vi "Begin.vi"(11 "Image Size":T1=enum."160x120") -> (0 "error out":errorcluster)   [LabVIEW 2011]
doc: "Called before other user functions, this VI is expected to open initial I/O refnums, load in file data, and do all program initialization. Notice that the <B>error out</B> terminal is simply used for data flow. Wiring it to other structures or subVIs ensures that this VI runs first."
uses:
  <vilib>/Rock Robotics/WPI/Camera/WPI_CameraImageSize.ctl
  <vilib>/Rock Robotics/WPI/Camera/WPI_CameraExposure Values.ctl
  <vilib>/Rock Robotics/WPI/Camera/WPI_CameraFrameRate.ctl
  <vilib>/Rock Robotics/WPI/Camera/WPI_CameraWhite Balance Values.ctl
  <vilib>/Rock Robotics/SystemInterfaces/DIO/FPGA_DIOPWMChannel.ctl
  <vilib>/Rock Robotics/SystemInterfaces/DIO/FPGA_DIOChannel.ctl
  <vilib>/Rock Robotics/WPI/Encoder/WPI_EncoderType.ctl
  <vilib>/Rock Robotics/SystemInterfaces/Typedef/FPGA_TypedefAnalogModule.ctl
  <vilib>/Rock Robotics/SystemInterfaces/AI/FPGA_AIChannel.ctl
  <vilib>/Rock Robotics/SystemInterfaces/Typedef/FPGA_TypedefDigitalModule.ctl
  <vilib>/Rock Robotics/SystemInterfaces/DIO/FPGA_DIORelayChannel.ctl
  <vilib>/Rock Robotics/WPI/Joystick/WPI_JoystickDeviceEnum.ctl
  <vilib>/Rock Robotics/SystemInterfaces/Typedef/FPGA_TypedefSolenoidModule.ctl
  <vilib>/Rock Robotics/WPI/Solenoid/WPI_SolenoidChannel.ctl
  <vilib>/Rock Robotics/WPI/Relay/WPI_RelayDirection.ctl
  <vilib>/Rock Robotics/WPI/RobotDrive/WPI_RobotDriveOpen4MotorWithVictor.vi
  <vilib>/Rock Robotics/WPI/MotorControl/WPI_MotorControlOpen Victor.vi
  <vilib>/Rock Robotics/WPI/Counter/WPI_CounterDigitalInputToDigitalSource.vi
  <vilib>/Rock Robotics/WPI/Counter/WPI_CounterOpen Gear Tooth Sensor Mode.vi
  <vilib>/Rock Robotics/WPI/Solenoid/WPI_SolenoidOpenDouble.vi
  <vilib>/Rock Robotics/WPI/Compressor/WPI_CompressorGetSetRefNum.vi
panel:
  in  "Image Size 2":T1=enum."160x120"
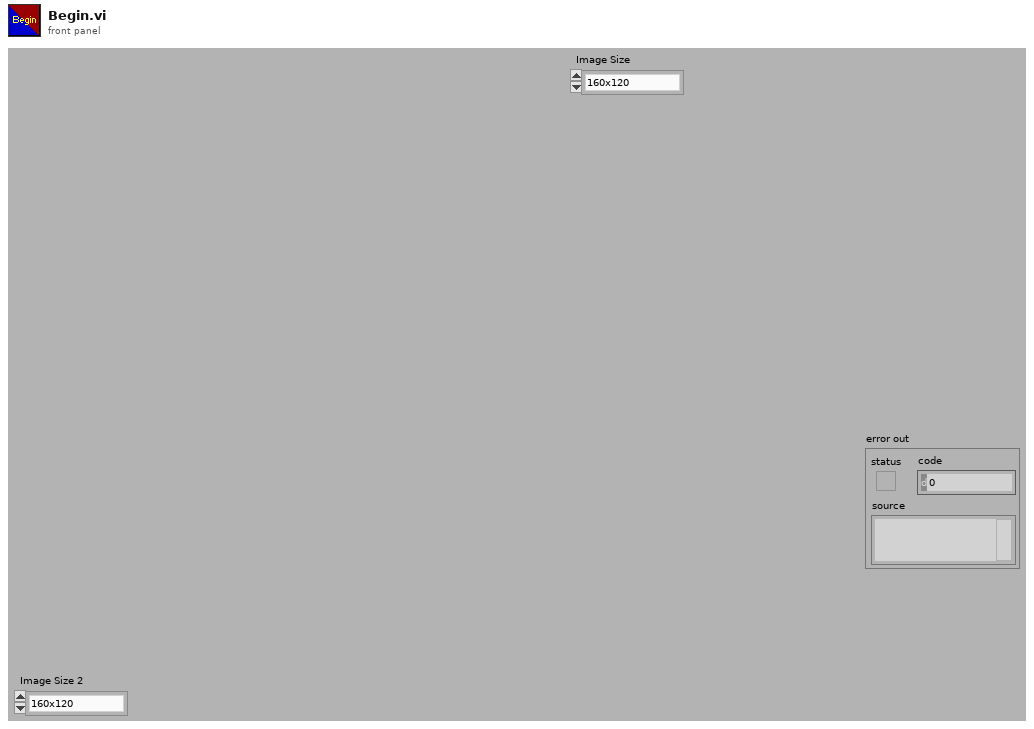
[diagram p1: front panel]
types:
  T1 = typedef "WPI_CameraImageSize.ctl" = enum16{"640x480", "320x240", "160x120"}
  T2 = typedef "WPI_RelayDirection.ctl" = enum16{"Both directions", "Forward only", "Reverse only"}
  T3 = typedef "FPGA_DIORelayChannel.ctl" = enum8{"Relay 1", "Relay 2", "Relay 3", "Relay 4", "Relay 5", "Relay 6", "Relay 7", "Relay 8", "Invalid"}
  T4 = typedef "FPGA_TypedefDigitalModule.ctl" = enum16{"Digital Module 1", "Digital Module 2"}
  T5 = typedef "WPI_SolenoidChannel.ctl" = enum8{"Solenoid 1", "Solenoid 2", "Solenoid 3", "Solenoid 4", "Solenoid 5", "Solenoid 6", "Solenoid 7", "Solenoid 8", "Invalid"}
  T6 = typedef "FPGA_TypedefSolenoidModule.ctl" = enum16{"Solenoid Module 1", "Solenoid Module 2"}
  T7 = typedef "FPGA_DIOChannel.ctl" = enum8{"DIO 1", "DIO 2", "DIO 3", "DIO 4", "DIO 5", "DIO 6", "DIO 7", "DIO 8", "DIO 9", "DIO 10", "DIO 11", "DIO 12", "DIO 13", "DIO 14", "Invalid"}
  T8 = typedef "WPI_JoystickDeviceEnum.ctl" = enum16{"USB 1", "USB 2", "USB 3", "USB 4", "Kinect 1", "Kinect 2"}
  T9 = typedef "FPGA_DIOPWMChannel.ctl" = enum8{"PWM 1", "PWM 2", "PWM 3", "PWM 4", "PWM 5", "PWM 6", "PWM 7", "PWM 8", "PWM 9", "PWM 10", "Invalid"}
  T10 = typedef "FPGA_AIChannel.ctl" = enum8{"AI 1", "AI 2", "AI 3", "AI 4", "AI 5", "AI 6", "AI 7", "AI 8", "Invalid"}
  T11 = typedef "FPGA_TypedefAnalogModule.ctl" = enum16{"Analog Module 1", "Analog Module 2"}
  T12 = typedef "WPI_EncoderType.ctl" = enum16{"1x", "2x", "4x"}
  T13 = typedef "WPI_CameraFrameRate.ctl" = u32
  T14 = typedef "WPI_CameraExposure Values.ctl" = enum16{"Auto", "Flicker-free 50 Hz", "Flicker-free 60 Hz", "Hold current"}
  T15 = typedef "WPI_CameraWhite Balance Values.ctl" = enum16{"Auto", "Fixed indoor", "Fixed outdoor 1", "Fixed outdoor 2", "Fixed fluorescent 1", "Fixed fluorescent 2", "Hold current"}
  T16 = typedef "WPI_MotorControlDeviceRef.ctl" = cluster{"DeviceStatus":errorcluster, "Type":enum16{"PWM", "CAN"}, "PWM":cluster{"Digital Module":T4, "PWM Channel":T9, "DeadBand":T17}, "CAN":cluster{"Device Number":u8, "Control Mode":T18, "Semaphore":T19, "Max Vout":dbl}, "Invert":bool, "TransformRef":T20, "InvTransformRef":T20}
  T17 = typedef "WPI_PWMDeadband.ctl" = cluster{"Name":string, "maxPositivePwm":i32, "minPositivePwm":i32, "centerPwm":i32, "maxNegativePwm":i32, "minNegativePwm":i32, "angularRange":u16}
  T18 = typedef "WPI_CANJaguar_ControlMode.ctl" = enum8{"Percent VBus", "Current", "Speed", "Position", "Voltage"}
  T19 = typedef "Semaphore RefNum" = refnum<k1>
  T20 = typedef "WPI_PWMTransform_ConPane.ctl" = refnum<vi>
  T21 = typedef "WPI_RobotDriveDevRef.ctl" = cluster{"DevStatus":errorcluster, "Motors[]":T16[], "Square Inputs":bool, "Max Output":dbl, "Isochronous":bool}
  T22 = typedef "WPI_CameraDevRef.ctl" = cluster{"Camera Address":string, "CameraStatus":errorcluster, "Acquire Image Notifier":refnum<notifier>}
  T23 = typedef "WPI_DigitalInputDevRef.ctl" = cluster{"DevStatus":errorcluster, "DIO Channel":T7, "Digital Module":T4}
  T24 = typedef "WPI_JoystickDevRef.ctl" = cluster{"Device":T8}
  T25 = typedef "WPI_AnalogChannelDevRef.ctl" = cluster{"DevStatus":errorcluster, "Analog Module":T11, "Analog Channel":T10}
  T26 = typedef "WPI_RelayDevRef.ctl" = cluster{"DevStatus":errorcluster, "Relay Channel":T3, "Digital Module":T4, "Relay Direction":T2}
  T27 = typedef "FPGA_CounterEncoderSourceConvertionLVSourceType.ctl" = cluster{"DevStatus":errorcluster, "AnalogTriggerMode?":bool, "DigitalMode":cluster{"Digital Module":T4, "DIO Channel":T28}, "AnalogTriggerMode":cluster{"AnalogTriggerIndex":T29, "OutputType":T30}}
  T28 = typedef "FPGA_DIODigitalSourceChannel.ctl" = enum8{"DIO 1", "DIO 2", "DIO 3", "DIO 4", "DIO 5", "DIO 6", "DIO 7", "DIO 8", "DIO 9", "DIO 10", "DIO 11", "DIO 12", "DIO 13", "DIO 14", "Disabled"}
  T29 = typedef "FPGA_AnalogTriggerIndex.ctl" = enum8{"Trig 0", "Trig 1", "Trig 2", "Trig 3", "Trig 4", "Trig 5", "Trig 6", "Trig 7", "Invalid"}
  T30 = typedef "FPGA_AnalogTriggerOutType.ctl" = enum16{"InWindow", "TriggerState", "Rising", "Falling"}
  T31 = typedef "WPI_EncoderDevRef.ctl" = cluster{"DevStatus":errorcluster, "EncoderIndex":T32, "CounterIndex":T33, "DistancePerCount":dbl, "Decoding Type":T12}
  T32 = typedef "FPGA_EncoderIdx.ctl" = enum8{"Enc 0", "Enc 1", "Enc 2", "Enc 3", "Invalid"}
  T33 = typedef "FPGA_CounterCtrSystemIndex.ctl" = enum8{"Ctr 0", "Ctr 1", "Ctr 2", "Ctr 3", "Ctr 4", "Ctr 5", "Ctr 6", "Ctr 7", "Invalid"}
  T34 = typedef "WPI_SolenoidDevRef.ctl" = cluster{"DevStatus":errorcluster, "Solenoid Module":T6, "Forward Solenoid Channel":T5, "Reverse Solenoid Channel":T5}
  T35 = typedef "WPI_CompressorDevRef.ctl" = cluster{"DevStatus":errorcluster, "DigitalInputDevRef":T23, "RelayDevRef":T26}
  T36 = typedef "WPI_CounterDevRef.ctl" = cluster{"DevStatus":errorcluster, "CntIndex":T33}
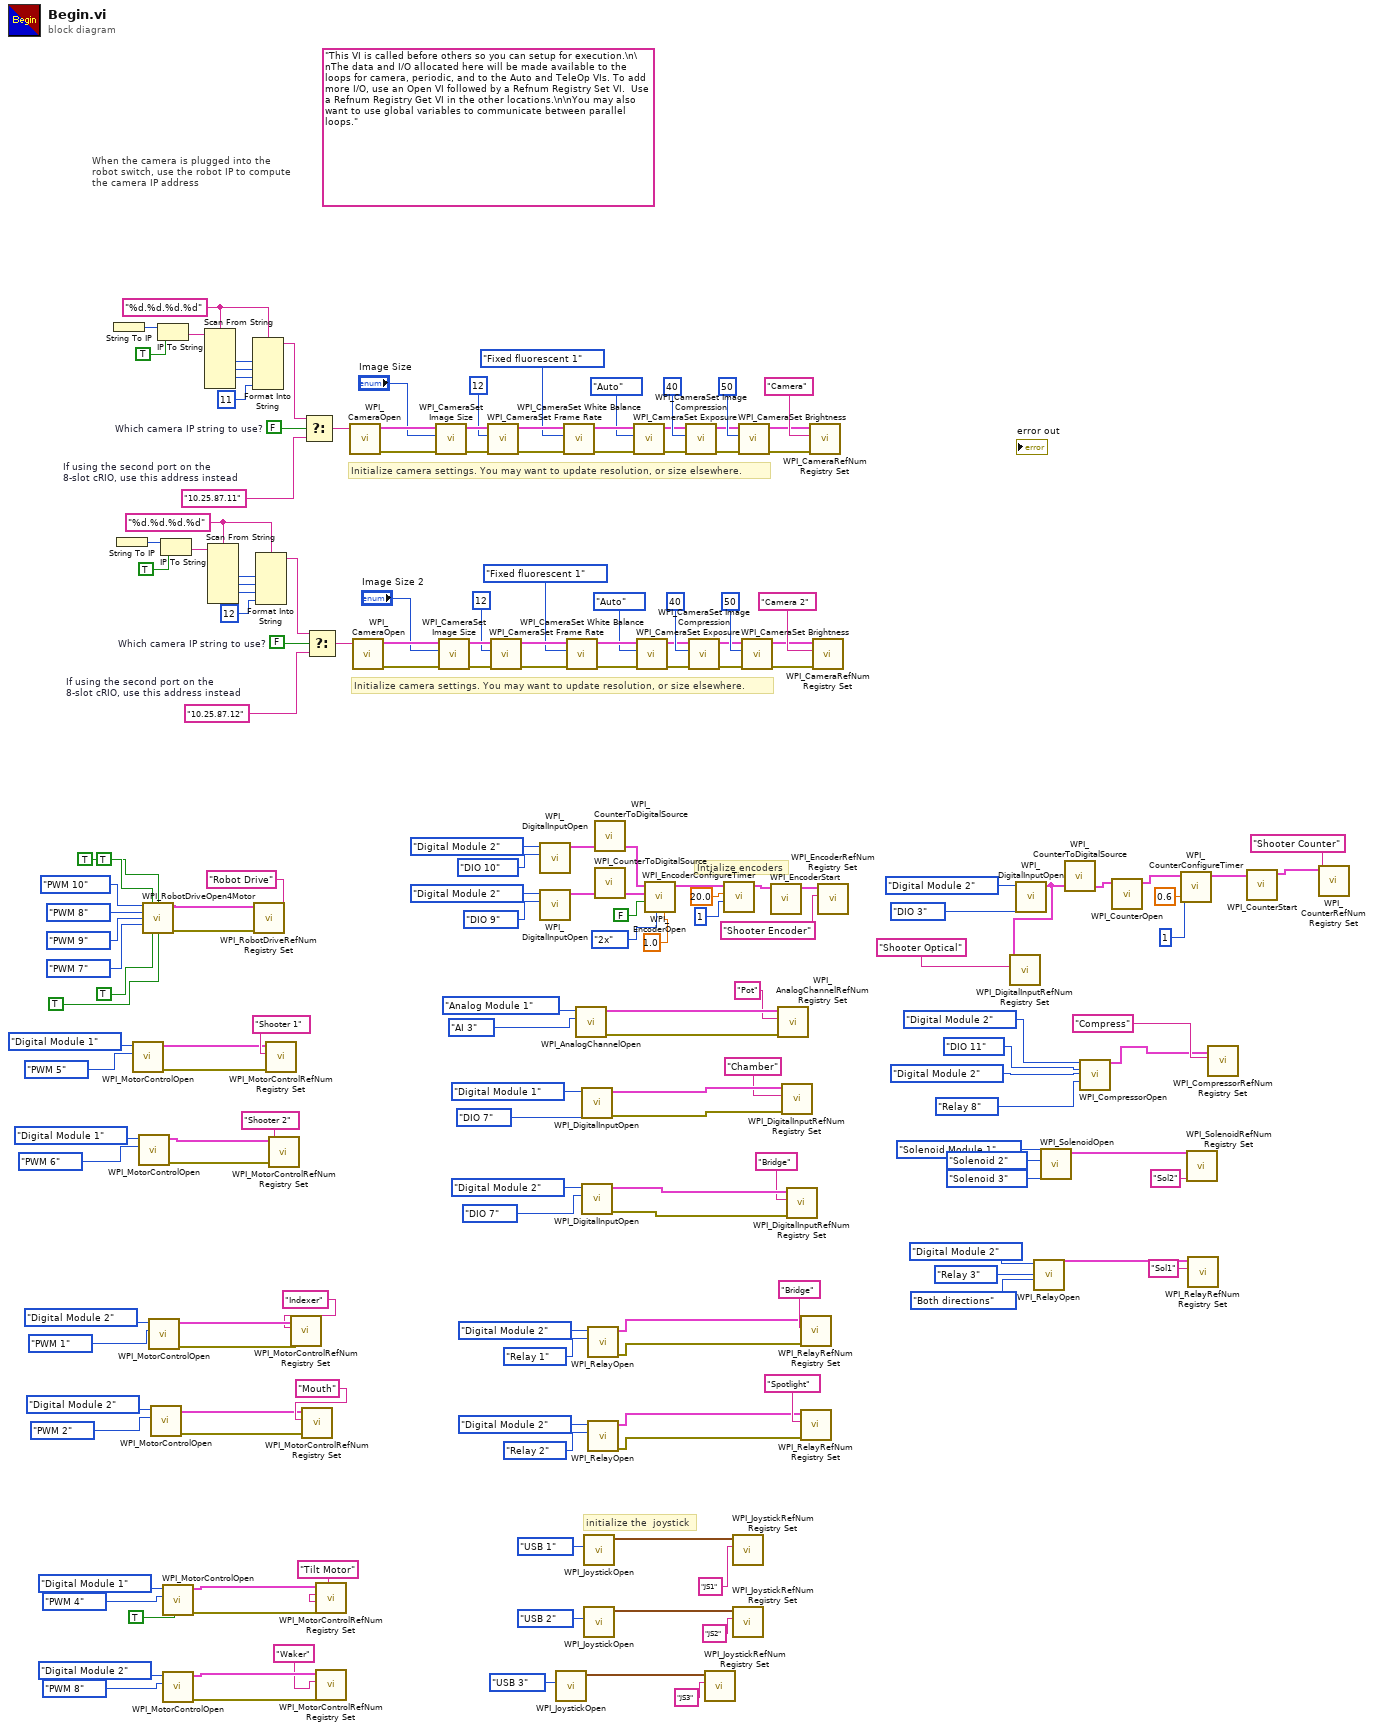
[diagram p0: block diagram]
diagram:
  w121 = FALSE  # Which camera IP string to use?
  w125 = "%d.%d.%d.%d" ("format string")
  w122 = "10.25.87.12"  # If using the second port on the 8-slot cRIO, use this address instead
  w154 = FALSE  # Which camera IP string to use?
  w158 = "%d.%d.%d.%d" ("format string")
  (unwired) "This VI is called before others so you can setup for execution.\n\nThe data and I/O allocated here will be made available to the loops for camera, periodic, and to the Auto and TeleOp VIs. To add more I/O, use an Open VI followed by a Refnum Registry Set VI.  Use a Refnum Registry Get VI in the other locations.\n\nYou may also want to use global variables to communicate between parallel loops."
  w155 = "10.25.87.11"  # If using the second port on the 8-slot cRIO, use this address instead
  # "initialize the  joystick"
  # "Intialize encoders"
  # "Initialize camera settings. You may want to update resolution, or size elsewhere."
  # "When the camera is plugged into the\nrobot switch, use the robot IP to compute\nthe camera IP address"
  # "Initialize camera settings. You may want to update resolution, or size elsewhere."
  n1 = String To IP() -> (0:w165:u32)  [unwired: 1 in]
  n2 = String To IP() -> (0:w132:u32)  [unwired: 1 in]
  n3 = call-poly <vilib>:"WPI_MotorControlOpen.vi"("PWM Channel"=FPGA_DIOPWMChannel."PWM 5", "Digital Module (Module 1)"=FPGA_TypedefDigitalModule."Digital Module 1") -> ("error out"=w104:errorcluster, "MotorControlDeviceRef"=w105:T16)  [unwired: 8 in]
  n4 = call-poly <vilib>:"WPI_MotorControlOpen.vi"("PWM Channel"=FPGA_DIOPWMChannel."PWM 6", "Digital Module (Module 1)"=FPGA_TypedefDigitalModule."Digital Module 1") -> ("error out"=w102:errorcluster, "MotorControlDeviceRef"=w103:T16)  [unwired: 8 in]
  n5 = call-poly <vilib>:"WPI_RobotDriveOpen4Motor.vi"("Rear Left Motor"=FPGA_DIOPWMChannel."PWM 10", "Rear Left Motor Inverted"=TRUE, "Rear Right Motor Inverted"=TRUE, "Rear Right Motor"=FPGA_DIOPWMChannel."PWM 8", "Front Left Motor"=FPGA_DIOPWMChannel."PWM 9", "Front Right Motor"=FPGA_DIOPWMChannel."PWM 7", "Front Left Motor Inverted"=TRUE, "Front Right Motor Inverted"=TRUE) -> ("RobotDriveDevRef"=w47:T21, "error out"=w46:errorcluster)  [unwired: 6 in]
  n6 = call-poly <vilib>:"WPI_MotorControlOpen.vi"("PWM Channel"=FPGA_DIOPWMChannel."PWM 1", "Digital Module (Module 1)"=FPGA_TypedefDigitalModule."Digital Module 2") -> ("error out"=w55:errorcluster, "MotorControlDeviceRef"=w56:T16)  [unwired: 8 in]
  n7 = call-poly <vilib>:"WPI_MotorControlOpen.vi"("PWM Channel"=FPGA_DIOPWMChannel."PWM 2", "Digital Module (Module 1)"=FPGA_TypedefDigitalModule."Digital Module 2") -> ("error out"=w97:errorcluster, "MotorControlDeviceRef"=w98:T16)  [unwired: 8 in]
  n8 = IP To String(1:TRUE ("dot notation? (F)"), 2:w165) -> (0:w163:string)
  n9 = IP To String(1:TRUE ("dot notation? (F)"), 2:w132) -> (0:w130:string)
  n10 = call-poly <vilib>:"WPI_MotorControlOpen.vi"("Invert"=TRUE, "PWM Channel"=FPGA_DIOPWMChannel."PWM 4", "Digital Module (Module 1)"=FPGA_TypedefDigitalModule."Digital Module 1") -> ("error out"=w91:errorcluster, "MotorControlDeviceRef"=w92:T16)  [unwired: 7 in]
  n11 = call-poly <vilib>:"WPI_MotorControlOpen.vi"("PWM Channel"=FPGA_DIOPWMChannel."PWM 8", "Digital Module (Module 1)"=FPGA_TypedefDigitalModule."Digital Module 2") -> ("error out"=w35:errorcluster, "MotorControlDeviceRef"=w34:T16)  [unwired: 8 in]
  n12 = Scan From String(format string=w158, input string=w163) -> (output 1=w162:i32, output 2=w161:i32, output 3=w160:i32)  [unwired: 7 in, 3 out]
  n13 = Scan From String(format string=w125, input string=w130) -> (output 1=w129:i32, output 2=w128:i32, output 3=w127:i32)  [unwired: 7 in, 3 out]
  n14 = Format Into String(format string=w158, w162, w161, w160, 11 ("Compression")) -> (resulting string=w156:string)  [unwired: 2 in, 1 out]
  n15 = call <vilib>:"WPI_RobotDriveRefNum Registry Set.vi"("error in (no error)"=w46, "refnum name"="Robot Drive", "RobotDriveDevRef"=w47) -> ()  [unwired: 7 in, 2 out]
  n16 = Format Into String(format string=w125, w129, w128, w127, 12 ("Compression")) -> (resulting string=w123:string)  [unwired: 2 in, 1 out]
  n17 = call <vilib>:"WPI_MotorControlRefNum Registry Set.vi"("error in (no error)"=w104, "refnum name"="Shooter 1", "MotorControlDevRef"=w105) -> ()  [unwired: 7 in, 2 out]
  n18 = call <vilib>:"WPI_MotorControlRefNum Registry Set.vi"("error in (no error)"=w102, "refnum name"="Shooter 2", "MotorControlDevRef"=w103) -> ()  [unwired: 7 in, 2 out]
  n19 = call <vilib>:"WPI_MotorControlRefNum Registry Set.vi"("error in (no error)"=w55, "refnum name"="Indexer", "MotorControlDevRef"=w56) -> ()  [unwired: 7 in, 2 out]
  n20 = call <vilib>:"WPI_MotorControlRefNum Registry Set.vi"("error in (no error)"=w97, "refnum name"="Mouth", "MotorControlDevRef"=w98) -> ()  [unwired: 7 in, 2 out]
  n21 = Select(t=w156, s=w154, f=w155) -> (s? t:f=w157:string)
  n22 = Select(t=w123, s=w121, f=w122) -> (s? t:f=w124:string)
  n23 = call <vilib>:"WPI_MotorControlRefNum Registry Set.vi"("error in (no error)"=w91, "refnum name"="Tilt Motor", "MotorControlDevRef"=w92) -> ()  [unwired: 7 in, 2 out]
  n24 = call <vilib>:"WPI_MotorControlRefNum Registry Set.vi"("error in (no error)"=w35, "refnum name"="Waker", "MotorControlDevRef"=w34) -> ()  [unwired: 7 in, 2 out]
  n25 = call <vilib>:"WPI_CameraOpen.vi"("Camera Address"=w157) -> ("error out"=w177:errorcluster, "CameraDevRef"=w178:T22)  [unwired: 1 in, 8 out]
  n26 = call <vilib>:"WPI_CameraOpen.vi"("Camera Address"=w124) -> ("error out"=w144:errorcluster, "CameraDevRef"=w145:T22)  [unwired: 1 in, 8 out]
  n27 = call <vilib>:"WPI_CameraSet Image Size.vi"("error in (no error)"=w177, "Image Size"="Image Size", "CameraDevRef"=w178) -> ("error out"=w176:errorcluster, "CameraDevRef Out"=w179:T22)  [unwired: 7 out]
  n28 = call <vilib>:"WPI_CameraSet Image Size.vi"("error in (no error)"=w144, "Image Size"="Image Size 2", "CameraDevRef"=w145) -> ("error out"=w143:errorcluster, "CameraDevRef Out"=w146:T22)  [unwired: 7 out]
  n29 = call <vilib>:"WPI_CameraSet Frame Rate.vi"("error in (no error)"=w176, "Frame Rate (fps)"=T13 12, "CameraDevRef"=w179) -> ("error out"=w175:errorcluster, "CameraDevRef Out"=w181:T22)  [unwired: 7 out]
  n30 = call <vilib>:"WPI_CameraSet Frame Rate.vi"("error in (no error)"=w143, "Frame Rate (fps)"=T13 12, "CameraDevRef"=w146) -> ("error out"=w142:errorcluster, "CameraDevRef Out"=w148:T22)  [unwired: 7 out]
  n31 = call <vilib>:"WPI_DigitalInputOpen.vi"("DIO Channel"=FPGA_DIOChannel."DIO 10", "Digital Module (Module 1)"=FPGA_TypedefDigitalModule."Digital Module 2") -> ("DigitalInputDevRef"=w88:T23)  [unwired: 8 in, 1 out]
  n32 = call <vilib>:"WPI_DigitalInputOpen.vi"("DIO Channel"=FPGA_DIOChannel."DIO 9", "Digital Module (Module 1)"=FPGA_TypedefDigitalModule."Digital Module 2") -> ("DigitalInputDevRef"=w84:T23)  [unwired: 8 in, 1 out]
  n33 = call <vilib>:"WPI_JoystickOpen.vi"("JoystickDevice"=WPI_JoystickDeviceEnum."USB 3") -> ("JoystickDevRef"=w19:T24)  [unwired: 10 out]
  n34 = call <vilib>:"WPI_CameraSet White Balance.vi"("error in (no error)"=w175, "White Balance"=WPI_CameraWhite_Balance_Values."Fixed fluorescent 1", "CameraDevRef"=w181) -> ("error out"=w174:errorcluster, "CameraDevRef Out"=w180:T22)  [unwired: 7 out]
  n35 = call <vilib>:"WPI_CameraSet White Balance.vi"("error in (no error)"=w142, "White Balance"=WPI_CameraWhite_Balance_Values."Fixed fluorescent 1", "CameraDevRef"=w148) -> ("error out"=w141:errorcluster, "CameraDevRef Out"=w147:T22)  [unwired: 7 out]
  n36 = call <vilib>:"WPI_AnalogChannelOpen.vi"("Analog Channel"=FPGA_AIChannel."AI 3", "Analog Module (Module 1)"=FPGA_TypedefAnalogModule."Analog Module 1") -> ("error out"=w69:errorcluster, "AIDeviceRef"=w71:T25)  [unwired: 8 in]
  n37 = call <vilib>:"WPI_DigitalInputOpen.vi"("DIO Channel"=FPGA_DIOChannel."DIO 7", "Digital Module (Module 1)"=FPGA_TypedefDigitalModule."Digital Module 1") -> ("error out"=w64:errorcluster, "DigitalInputDevRef"=w66:T23)  [unwired: 8 in]
  n38 = call <vilib>:"WPI_DigitalInputOpen.vi"("DIO Channel"=FPGA_DIOChannel."DIO 7", "Digital Module (Module 1)"=FPGA_TypedefDigitalModule."Digital Module 2") -> ("error out"=w36:errorcluster, "DigitalInputDevRef"=w38:T23)  [unwired: 8 in]
  n39 = call <vilib>:"WPI_JoystickOpen.vi"("JoystickDevice"=WPI_JoystickDeviceEnum."USB 1") -> ("JoystickDevRef"=w51:T24)  [unwired: 10 out]
  n40 = call <vilib>:"WPI_JoystickOpen.vi"("JoystickDevice"=WPI_JoystickDeviceEnum."USB 2") -> ("JoystickDevRef"=w50:T24)  [unwired: 10 out]
  n41 = call <vilib>:"WPI_RelayOpen.vi"("Relay Channel"=FPGA_DIORelayChannel."Relay 1", "Digital Module (Module 1)"=FPGA_TypedefDigitalModule."Digital Module 2") -> ("error out"=w41:errorcluster, "RelayDevRef"=w42:T26)  [unwired: 8 in]
  n42 = call <vilib>:"WPI_RelayOpen.vi"("Relay Channel"=FPGA_DIORelayChannel."Relay 2", "Digital Module (Module 1)"=FPGA_TypedefDigitalModule."Digital Module 2") -> ("error out"=w59:errorcluster, "RelayDevRef"=w60:T26)  [unwired: 8 in]
  n43 = call-poly <vilib>:"WPI_CounterToDigitalSource.vi"("DigitalInputDevRef"=w88) -> ("Digital Source"=w87:T27)  [unwired: 6 in]
  n44 = call-poly <vilib>:"WPI_CounterToDigitalSource.vi"("DigitalInputDevRef"=w84) -> ("Digital Source"=w83:T27)  [unwired: 6 in]
  n45 = call <vilib>:"WPI_CameraSet Exposure.vi"("error in (no error)"=w174, "Exposure"=WPI_CameraExposure_Values."Auto", "CameraDevRef"=w180) -> ("error out"=w173:errorcluster, "CameraDevRef Out"=w183:T22)  [unwired: 7 out]
  n46 = call <vilib>:"WPI_CameraSet Exposure.vi"("error in (no error)"=w141, "Exposure"=WPI_CameraExposure_Values."Auto", "CameraDevRef"=w147) -> ("error out"=w140:errorcluster, "CameraDevRef Out"=w150:T22)  [unwired: 7 out]
  n47 = call <vilib>:"WPI_EncoderOpen.vi"("DistancePerCount"=1.0, "Decoding Type"=WPI_EncoderType."2x", "Invert Direction (False)"=FALSE, "BSource"=w83, "ASource"=w87) -> ("EncoderDevRef"=w81:T31)  [unwired: 5 in, 1 out]
  n48 = call <vilib>:"WPI_CameraSet Image Compression.vi"("error in (no error)"=w173, "Compression"=40, "CameraDevRef"=w183) -> ("error out"=w172:errorcluster, "CameraDevRef Out"=w182:T22)  [unwired: 7 out]
  n49 = call <vilib>:"WPI_CameraSet Image Compression.vi"("error in (no error)"=w140, "Compression"=40, "CameraDevRef"=w150) -> ("error out"=w139:errorcluster, "CameraDevRef Out"=w149:T22)  [unwired: 7 out]
  n50 = call <vilib>:"WPI_JoystickRefNum Registry Set.vi"("refnum name"="JS3", "JoystickDevRef"=w19) -> ()  [unwired: 1 in, 9 out]
  n51 = call <vilib>:"WPI_EncoderConfigureTimer.vi"("Number Samples to Average"=u8 1, "Minimum Rate"=20.0, "EncoderDevRef"=w81) -> ("EncoderDevRef"=w75:T31)  [unwired: 7 in, 1 out]
  n52 = call <vilib>:"WPI_JoystickRefNum Registry Set.vi"("refnum name"="JS1", "JoystickDevRef"=w51) -> ()  [unwired: 1 in, 9 out]
  n53 = call <vilib>:"WPI_JoystickRefNum Registry Set.vi"("refnum name"="JS2", "JoystickDevRef"=w50) -> ()  [unwired: 1 in, 9 out]
  n54 = call <vilib>:"WPI_CameraSet Brightness.vi"("error in (no error)"=w172, "Brightness"=50, "CameraDevRef"=w182) -> ("error out"=w170:errorcluster, "CameraDevRef Out"=w171:T22)  [unwired: 7 out]
  n55 = call <vilib>:"WPI_CameraSet Brightness.vi"("error in (no error)"=w139, "Brightness"=50, "CameraDevRef"=w149) -> ("error out"=w137:errorcluster, "CameraDevRef Out"=w138:T22)  [unwired: 7 out]
  n56 = call <vilib>:"WPI_EncoderStart.vi"("EncoderDevRef"=w75) -> ("EncoderDevRef"=w74:T31)  [unwired: 9 in, 1 out]
  n57 = call <vilib>:"WPI_AnalogChannelRefNum Registry Set.vi"("error in (no error)"=w69, "refnum name"="Pot", "AIDeviceRef"=w71) -> ()  [unwired: 7 in, 2 out]
  n58 = call <vilib>:"WPI_DigitalInputRefNum Registry Set.vi"("error in (no error)"=w64, "refnum name"="Chamber", "DigitalInputDevRef"=w66) -> ()  [unwired: 7 in, 2 out]
  n59 = call <vilib>:"WPI_DigitalInputRefNum Registry Set.vi"("error in (no error)"=w36, "refnum name"="Bridge", "DigitalInputDevRef"=w38) -> ()  [unwired: 7 in, 2 out]
  n60 = call <vilib>:"WPI_RelayRefNum Registry Set.vi"("error in (no error)"=w41, "refnum name"="Bridge", "RelayDevRef"=w42) -> ()  [unwired: 7 in, 2 out]
  n61 = call <vilib>:"WPI_RelayRefNum Registry Set.vi"("error in (no error)"=w59, "refnum name"="Spotlight", "RelayDevRef"=w60) -> ()  [unwired: 7 in, 2 out]
  n62 = call <vilib>:"WPI_CameraRefNum Registry Set.vi"("error in (no error)"=w170, "refnum name"="Camera", "CameraDevRef"=w171) -> ()  [unwired: 9 out]
  n63 = call <vilib>:"WPI_CameraRefNum Registry Set.vi"("error in (no error)"=w137, "refnum name"="Camera 2", "CameraDevRef"=w138) -> ()  [unwired: 9 out]
  n64 = call <vilib>:"WPI_EncoderRefNum Registry Set.vi"("refnum name"="Shooter Encoder", "EncoderDevRef"=w74) -> ()  [unwired: 8 in, 2 out]
  n65 = call <vilib>:"WPI_DigitalInputOpen.vi"("DIO Channel"=FPGA_DIOChannel."DIO 3", "Digital Module (Module 1)"=FPGA_TypedefDigitalModule."Digital Module 2") -> ("DigitalInputDevRef"=w27:T23)  [unwired: 8 in, 1 out]
  n66 = call <vilib>:"WPI_DigitalInputRefNum Registry Set.vi"("refnum name"="Shooter Optical", "DigitalInputDevRef"=w27) -> ()  [unwired: 8 in, 2 out]
  n67 = call <vilib>:"WPI_RelayOpen.vi"("Relay Direction"=WPI_RelayDirection."Both directions", "Relay Channel"=FPGA_DIORelayChannel."Relay 3", "Digital Module (Module 1)"=FPGA_TypedefDigitalModule."Digital Module 2") -> ("RelayDevRef"=w5:T26)  [unwired: 7 in, 1 out]
  n68 = call-poly <vilib>:"WPI_SolenoidOpen.vi"("Reverse Solenoid Channel"=WPI_SolenoidChannel."Solenoid 3", "Forward Solenoid Channel"=WPI_SolenoidChannel."Solenoid 2", "Solenoid Module (Module 1)"=FPGA_TypedefSolenoidModule."Solenoid Module 1") -> ("SolenoidDevRef"=w10:T34)  [unwired: 7 in, 1 out]
  n69 = call-poly <vilib>:"WPI_CounterToDigitalSource.vi"("DigitalInputDevRef"=w27) -> ("Digital Source"=w26:T27)  [unwired: 6 in]
  n70 = call <vilib>:"WPI_CompressorOpen.vi"("Pressure Switch Digital Module (Module 1)"=FPGA_TypedefDigitalModule."Digital Module 2", "Pressure Switch DIO Channel"=FPGA_DIOChannel."DIO 11", "Relay Digital Module (Module 1)"=FPGA_TypedefDigitalModule."Digital Module 2", "Relay Channel"=FPGA_DIORelayChannel."Relay 8") -> ("CompressorDevRef"=w11:T35)  [unwired: 10 in, 1 out]
  n71 = call-poly <vilib>:"WPI_CounterOpen.vi"("Source"=w26) -> ("CounterDevRef"=w22:T36)  [unwired: 9 in, 1 out]
  n72 = call <vilib>:"WPI_CounterConfigureTimer.vi"("Number Samples to Average"=u8 1, "MaxPeriod (sec)"=0.6, "CounterDevRef in"=w22) -> ("CounterDevRef out"=w24:T36)  [unwired: 7 in, 1 out]
  n73 = call <vilib>:"WPI_SolenoidRefNum Registry Set.vi"("refnum name"="Sol2", "SolenoidDevRef"=w10) -> ()  [unwired: 8 in, 2 out]
  n74 = call <vilib>:"WPI_RelayRefNum Registry Set.vi"("refnum name"="Sol1", "RelayDevRef"=w5) -> ()  [unwired: 8 in, 2 out]
  n75 = call <vilib>:"WPI_CompressorRefNum Registry Set.vi"("refnum name"="Compress", "CompressorDevRef"=w11) -> ()  [unwired: 8 in, 2 out]
  n76 = call <vilib>:"WPI_CounterStart.vi"("CounterDevRef in"=w24) -> ("CounterDevRef out"=w23:T36)  [unwired: 9 in, 1 out]
  n77 = call <vilib>:"WPI_CounterRefNum Registry Set.vi"("refnum name"="Shooter Counter", "CounterDevRef"=w23) -> ()  [unwired: 8 in, 2 out]
